vi "Exception Handler.vi"() -> ()   [LabVIEW 2020, in "Startup Processes.lvlib"]
uses:
  Startup Processes.lvlib
  toolbox/Standard Signalling/ude_Stop Application/ude_Stop Application.lvlib
  toolbox/Standard Signalling/ude_Handle Errors/ude_Handle Errors.lvlib
  toolbox/Error Reporting and Storage/Error Reporting and Storage.lvlib
  toolbox/Timing/Timing.lvlib
  Config Data/Config Data.lvclass
panel:
  in  "Stop Button":bool
  out "Last Error Reported":errorcluster
  # "This VI has no user interface...."
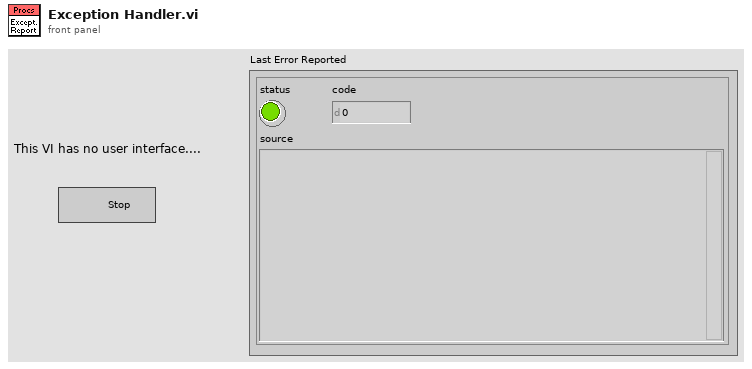
[diagram p1: front panel]
types:
  T1 = cluster{"sys":refnum<event-registration>, "sys":refnum<event-registration>}
  T2 = enum16{"Ok + Logging", "Continue/Stop + Logging", "Logging Only", "Ok Only", "Continue/Stop Only"}
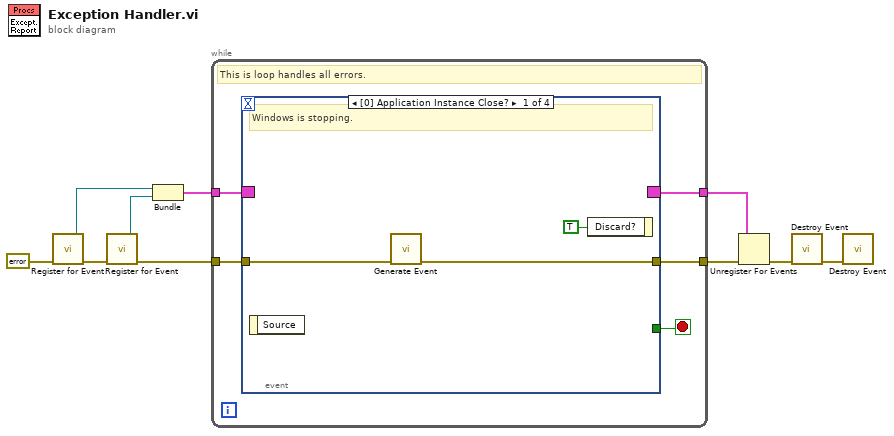
[diagram p0: block diagram]
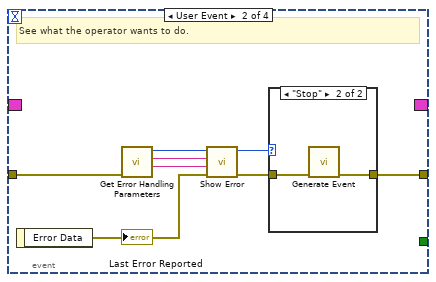
[diagram p2: hidden frame]
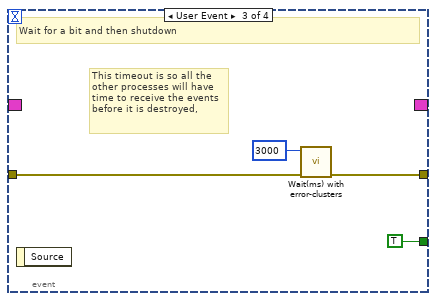
[diagram p4: hidden frame]
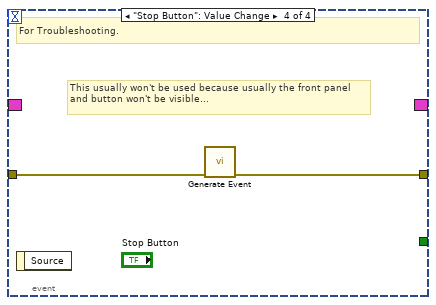
[diagram p5: hidden frame]
diagram:
  n1 = call "Register for Event.vi"("Error In"=errorcluster {"status"=FALSE, "code"=0, "source"=""}) -> ("Error Out"=w4:errorcluster, "sys"=w3:refnum<event-registration>)  [unwired: 5 in]
  n2 = call "Register for Event.vi"("Error In"=w4) -> ("Error Out"=w10:errorcluster, "sys"=w9:refnum<event-registration>)  [unwired: 5 in]
  n3 = Bundle("sys"=w3, "sys"=w9) -> (w8:T1)  [unwired: 1 in]
  n4 = while {
    tunnel: w8 -> [w15]
    tunnel: w10 -> [w14]
    tunnel: [w13] -> w6
    tunnel: [w12] -> w7
    stop <- w11 stop-if-true
    # "This is loop handles all errors."
    n5 = event shown="[0] Application Instance Close?" {
      selector: w15 -> [_ _ _ _]
      dyn-events: [_ _ _ _] -> w12
      timeout: _ -> [_ _ _ _]
      tunnel: w14 -> [w17 w22 w31 w35]
      tunnel: [w16 w26 w30 w34] -> w13
      tunnel: [_ _ TRUE _] -> w11
      event Application Instance Close? {
        # "Windows is stopping."
        n6 = event-data() -> ()  [unwired: 1 in, 1 out]
        n7 = call "Generate Event.vi"("Error In"=w17) -> ("Error Out"=w16:errorcluster)  [unwired: 6 in]
        n8 = event-data("Discard?"=TRUE) -> ()  [unwired: 1 in, 1 out]
      }
      event User Event {
        # "See what the operator wants to do."
        n9 = event-data() -> ("Error Data"=w25:errorcluster)  [unwired: 1 in]
        "Last Error Reported" <- w25
        n10 = call "Get Error Handling Parameters.vi"("Error In"=w22) -> ("Stop Button"=w19:string, "Continue/Ok Button"=w20:string, "Action"=w21:T2)  [unwired: 3 in, 1 out]
        n11 = call "Show Error.vi"("Error In"=w25, "Stop Button"=w19, "Continue/Ok Button"=w20, "Action"=w21) -> ("error out"=w24:errorcluster, "What's Next"=w23:enum16{"Continue", "Stop"})  [unwired: 2 in]
        n12 = case shown="\"Stop\"" w23 {
          tunnel: [w27 w29] -> w26
          tunnel: w24 -> [w27 w28]
          frame "Continue" {
          }
          frame "Stop" {
            n13 = call "Generate Event.vi"("Error In"=w28) -> ("Error Out"=w29:errorcluster)  [unwired: 6 in]
          }
        }
      }
      event User Event {
        # "This timeout is so all the other processes will have time to receive the events before it is destroyed,"
        # "Wait for a bit and then shutdown"
        n14 = event-data() -> ()  [unwired: 1 in, 1 out]
        n15 = call "Wait(ms) with error-clusters.vi"("Error In"=w31, "wait (msec)"=u32 3000 ("milliseconds to wait")) -> ("Error Out"=w30:errorcluster)  [unwired: 5 in]
      }
      event "Stop Button": Value Change {
        # "This usually won't be used because usually the front panel and button won't be visible..."
        # "For Troubleshooting."
        n16 = event-data() -> ()  [unwired: 1 in, 1 out]
        n17 = call "Generate Event.vi"("Error In"=w35) -> ("Error Out"=w34:errorcluster)  [unwired: 6 in]
      }
    }
  }
  n18 = Unregister For Events(event registration refnum=w7, error in=w6) -> (error out=w5:errorcluster)
  n19 = call "Destroy Event.vi"("Error In"=w5) -> ("Error Out"=w2:errorcluster)  [unwired: 6 in]
  n20 = call "Destroy Event.vi"("Error In"=w2) -> ()  [unwired: 6 in, 1 out]
